vi "Get Pixel Brightness.vi"(9 "B":u8, 10 "G":u8, 11 "R":u8) -> (3 "Brightness":dbl)   [LabVIEW 2015]
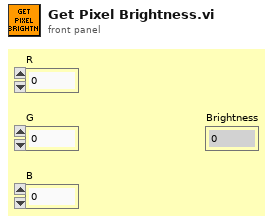
[diagram p1: front panel]
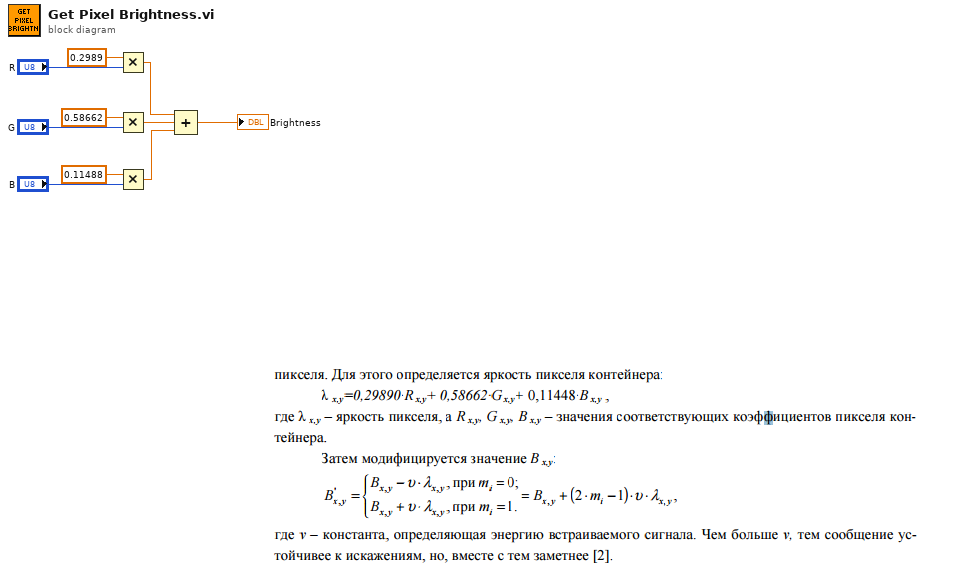
[diagram p0: block diagram]
diagram:
  n1 = Multiply(x=0.2989, y="R") -> (x*y=w4:dbl)
  n2 = Multiply(x=0.58662, y="G") -> (x*y=w3:dbl)
  n3 = Multiply(x=0.11488, y="B") -> (x*y=w2:dbl)
  n4 = Compound Arithmetic op=ADD(w4, w3, w2) -> (→"Brightness":dbl)
